vi "COBS Stuff.vi"(8 "error in (no error)":errorcluster, 11 "Raw Array in":u8[](array[numeric])) -> (0 "error out":errorcluster, 3 "Stuffed Array out":u8[](array[numeric]))   [LabVIEW 2015, in "LSR Transmission.lvlib"]
uses:
  LSR Transmission.lvlib
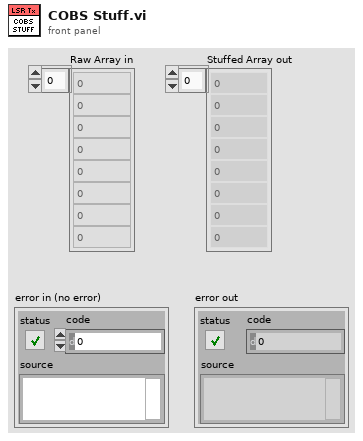
[diagram p1: front panel]
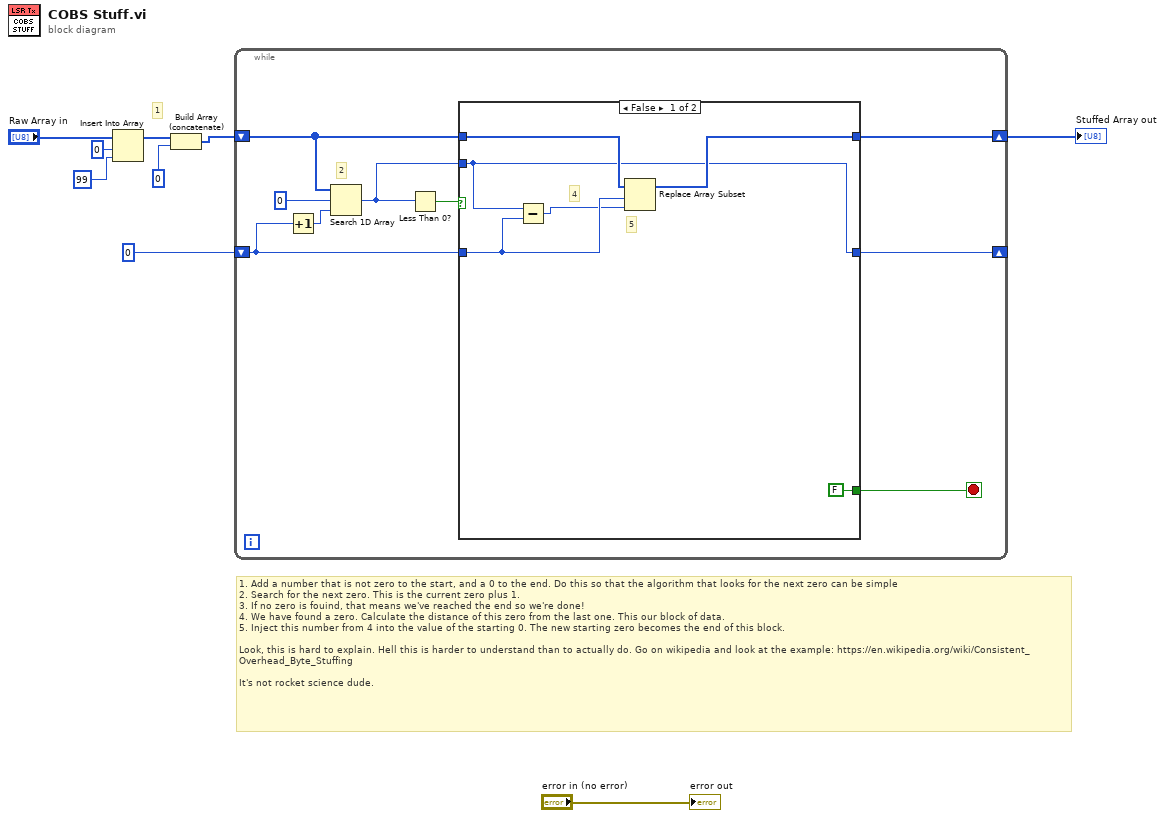
[diagram p0: block diagram]
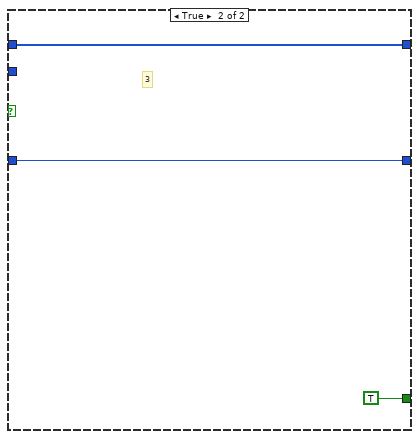
[diagram p2: hidden frame]
diagram:
  # "1. Add a number that is not zero to the start, and a 0 to the end. Do this so that the algorithm that looks for the next zero can be simple\n2. Search for the next zero. This is the current zero plus 1. \n3. If no zero is fouind, that means we've reached the end so we're done!\n4. We have found a zero. Calculate the distance of this zero from the last one. This our block of data.\n5. Inject this number from 4 into the value of the starting 0. The new starting zero becomes the end of this block.\n\nLook, this is hard to explain. Hell this is harder to understand than to actually do. Go on wikipedia and look at the example: https://en.wikipedia.org/wiki/Consistent_Overhead_Byte_Stuffing\n\nIt's not rocket science dude."
  # "1"
  n1 = Insert Into Array(array="Raw Array in", index=0, new element=u8 99 ("element")) -> (w7:u8[])
  n2 = Build Array (concatenate)(w7, u8 0 ("element")) -> (w8:u8[])
  n3 = while {
    shift-right: [w10] -> w1
    shift-left: w8 -> [w17]
    shift-right: [w14] -> _
    shift-left: u8 0 ("element") -> [w11]
    stop <- w16 stop-if-true
    # "2"
    n4 = Increment(x=w11) -> (x+1=w12:i32)
    n5 = Search 1D Array(1D array=w17, element=u8 0, start index (0)=w12) -> (index of element=w13:i32)
    n6 = Less Than 0?(x=w13) -> (x < 0?=w15:bool)
    n7 = case shown="False" w15 {
      tunnel: [w20 w25] -> w10
      tunnel: w17 -> [w21 w25]
      tunnel: [FALSE TRUE] -> w16
      tunnel: w11 -> [w23 w26]
      tunnel: [w19 w26] -> w14
      tunnel: w13 -> [w19 _]
      frame False {
        # "5"
        # "4"
        n8 = Subtract(x=w19, y=w23) -> (x-y=w22:i32)
        n9 = Replace Array Subset(array=w21, new element=w22, index=w23) -> (w20:u8[])
      }
      frame True {
        # "3"
      }
    }
  }
  "Stuffed Array out" <- w1
  "error out" <- "error in (no error)"
